vi "实时监测图放大.vi"() -> ()   [LabVIEW 2018]
panel:
  out "实时监测":cluster{"Value":timestamp[], "Value":dbl[]}[](graph)
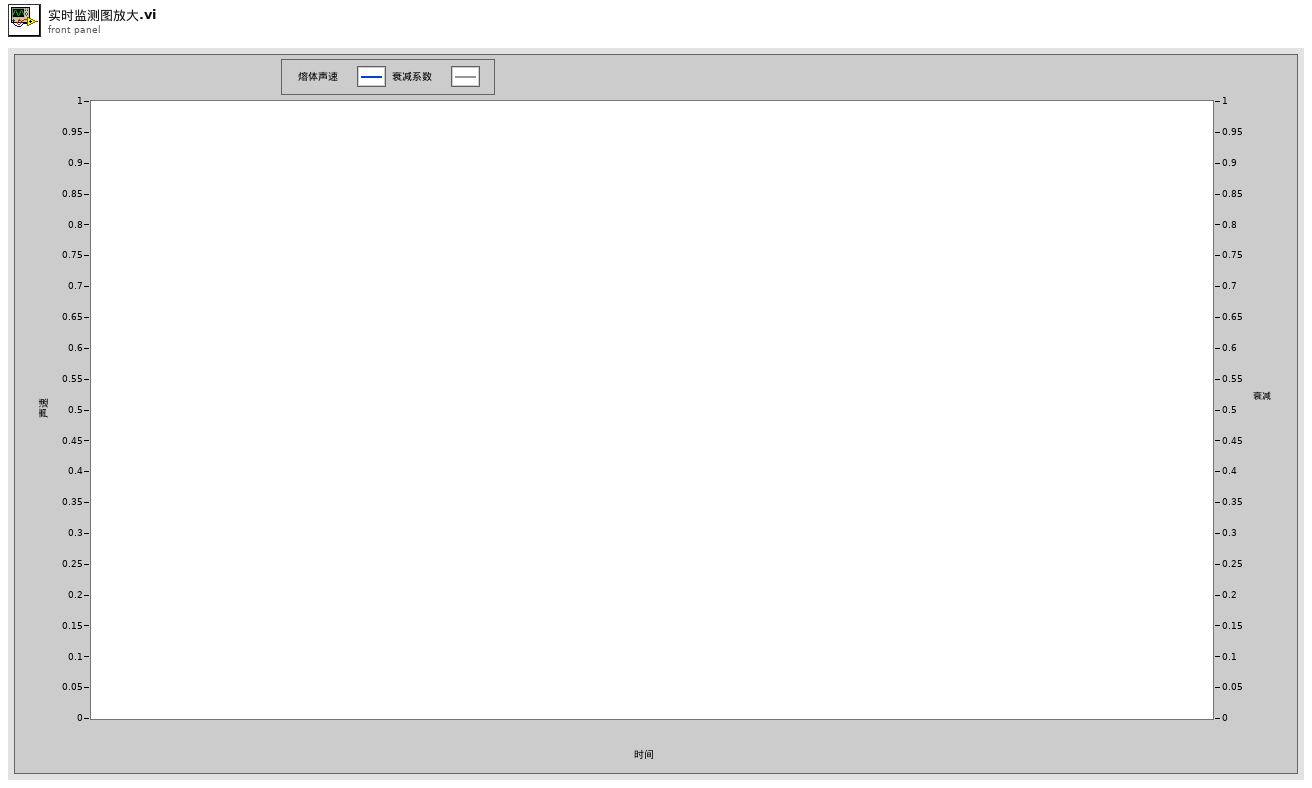
[diagram p1: front panel]
types:
  T1 = enum32{"Invalid", "Standard", "Closed", "Hidden", "Minimized", "Maximized"}
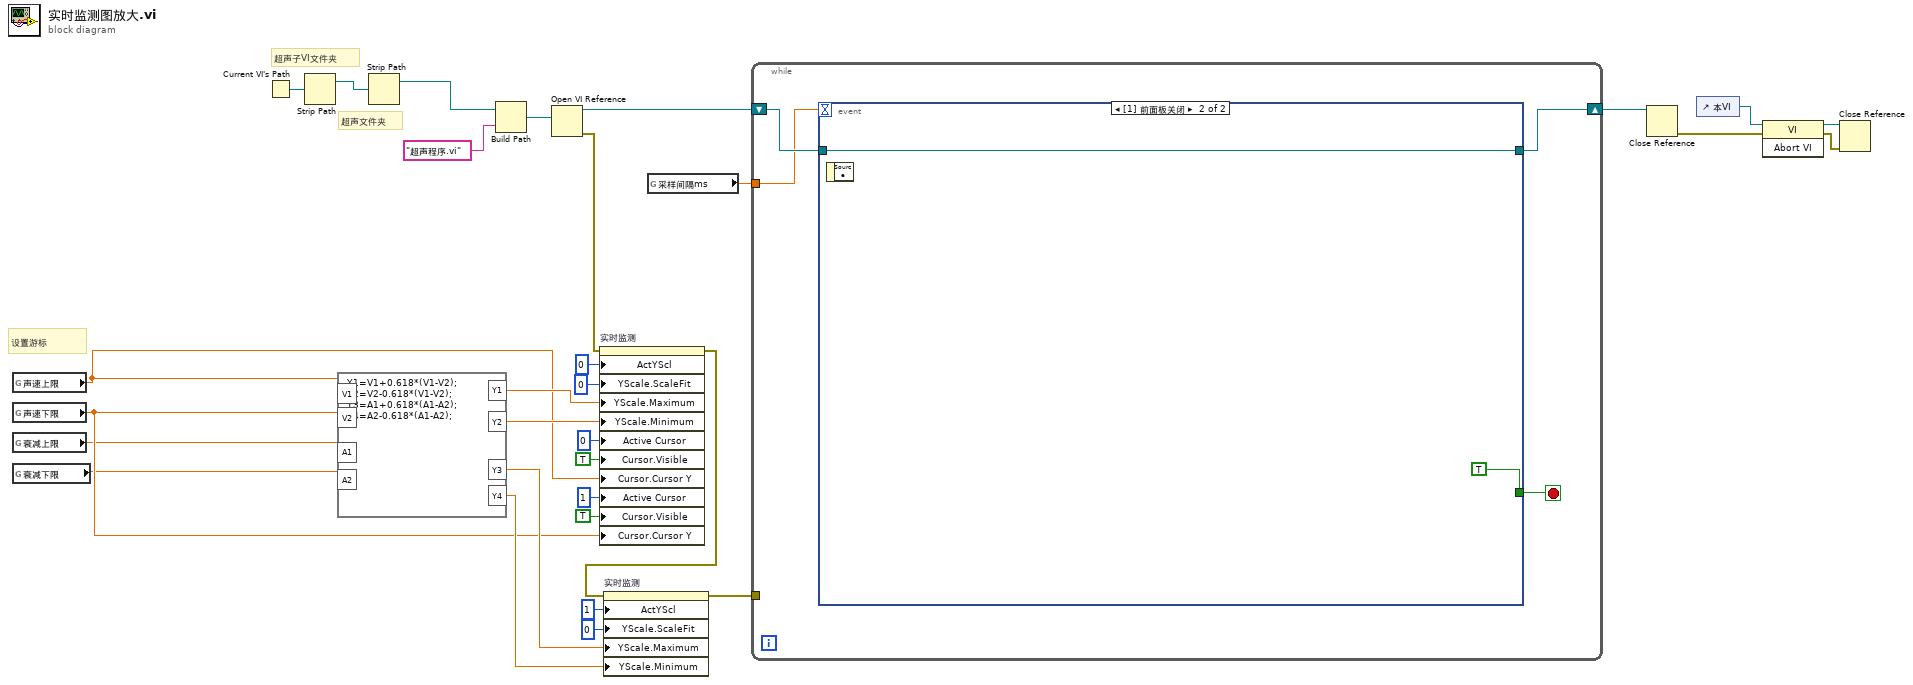
[diagram p0: block diagram]
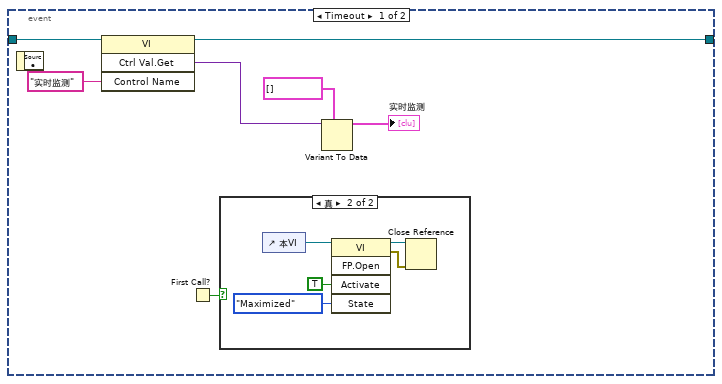
[diagram p2: hidden frame]
diagram:
  # "设置游标"
  # "超声文件夹"
  # "超声子VI文件夹"
  n1 = global read "超声_gbl.vi" "声速上限"() -> (w7:dbl)
  n2 = global read "超声_gbl.vi" "声速下限"() -> (w6:dbl)
  n3 = global read "超声_gbl.vi" "衰减上限"() -> (w5:dbl)
  n4 = global read "超声_gbl.vi" "衰减下限"() -> (w4:dbl)
  n5 = Current VI's Path() -> (path=w28:path)
  n6 = Strip Path(path=w28) -> (stripped path=w29:path)  [unwired: 1 out]
  n7 = formula code="Y1=V1+0.618*(V1-V2);\nY2=V2-0.618*(V1-V2);\nY3=A1+0.618*(A1-A2);\nY4=A2-0.618*(A1-A2);"("V1"=w7, "V2"=w6, "A1"=w5, "A2"=w4) -> ("Y1"=w17:dbl, "Y2"=w16:dbl, "Y3"=w11:dbl, "Y4"=w10:dbl)
  n8 = Strip Path(path=w29) -> (stripped path=w22:path)  [unwired: 1 out]
  n9 = Build Path(base path=w22, name or relative path="超声程序.vi" ("名称或相对路径")) -> (appended path=w31:path)
  n10 = Open VI Reference(vi path=w31) -> (vi reference=w21:refnum<vi>, error out=w1:errorcluster)  [unwired: 5 in]
  n11 = property on="实时监测" class="XYGraph (严格)"(error in=w1, "ActYScl"=0 ("活动Y标尺"), "YScale.ScaleFit"=u8 0 ("Y标尺.标尺调节"), "YScale.Maximum"=w17, "YScale.Minimum"=w16, "Active Cursor"=u32 0 ("活动游标"), "Cursor.Visible"=TRUE ("游标.可见"), "Cursor.Cursor Y"=w7, "Active Cursor"=u32 1 ("活动游标"), "Cursor.Visible"=TRUE ("游标.可见"), "Cursor.Cursor Y"=w6) -> (error out=w3:errorcluster)  [unwired: 1 in, 1 out]
  n12 = property on="实时监测" class="XYGraph (严格)"(error in=w3, "ActYScl"=1 ("活动Y标尺"), "YScale.ScaleFit"=u8 0 ("Y标尺.标尺调节"), "YScale.Maximum"=w11, "YScale.Minimum"=w10) -> (error out=w2:errorcluster)  [unwired: 1 in, 1 out]
  n13 = global read "超声_gbl.vi" "采样间隔ms"() -> (w20:dbl)
  n14 = while {
    shift-right: [w35] -> w27
    shift-left: w21 -> [w33]
    tunnel: w20 -> [w32]
    tunnel: w2 -> [_]
    stop <- w34 stop-if-true
    n15 = event shown="[1] 前面板关闭" {
      selector: _ -> [_ _]
      dyn-events: _ -> [_ _]
      timeout: w32 -> [_ _]
      tunnel: [w38 w49] -> w35
      tunnel: w33 -> [w41 w49]
      tunnel: [_ TRUE] -> w34
      event Timeout {
        n16 = event-data() -> ()  [unwired: 1 in, 1 out]
        n17 = invoke class="VI" method="Ctrl Val.Get"(reference=w41, "Control Name"="实时监测" ("控件名")) -> (reference out=w38:refnum<vi>, "Get Control Value Variant"=w40:variant)  [unwired: 2 in, 2 out]
        n18 = First Call?() -> (First Call?: T/F=w39:bool)
        n19 = case shown="真" w39 {
          frame False {
          }
          frame True {
            n20 = control-ref of="本VI"() -> (w47:refnum<vi>)
            n21 = invoke class="VI" method="FP.Open"(reference=w47, "Activate"=TRUE ("激活？"), "State"=T1."Maximized" ("状态")) -> (reference out=w43:refnum<vi>, error out=w44:errorcluster)  [unwired: 2 in, 3 out]
            n22 = Close Reference(reference=w43, error in (no error)=w44) -> ()  [unwired: 1 out]
          }
        }
        n23 = Variant To Data(type=cluster{"Value":timestamp[], "Value":dbl[]}[] [] ("XY图"), Variant=w40) -> (data=→"实时监测":cluster{"Value":timestamp[], "Value":dbl[]}[])  [unwired: 1 in, 1 out]
      }
      event Panel Close {
        n24 = event-data() -> ()  [unwired: 1 in, 1 out]
      }
    }
  }
  n25 = Close Reference(reference=w27) -> (error out=w25:errorcluster)  [unwired: 1 in]
  n26 = control-ref of="本VI"() -> (w26:refnum<vi>)
  n27 = invoke class="VI" method="Abort VI"(reference=w26, error in=w25) -> (reference out=w23:refnum<vi>, error out=w24:errorcluster)  [unwired: 1 in, 1 out]
  n28 = Close Reference(reference=w23, error in (no error)=w24) -> ()  [unwired: 1 out]
